vi "DataTreeCtrl unMountFile.vi"(8 "error in (no error)":errorcluster, 11 "DataTreeCtrl in":refnum<class "DataTreeCtrl.lvclass">) -> (0 "error out":errorcluster, 3 "DataTreeCtrl out":refnum<class "DataTreeCtrl.lvclass">)   [LabVIEW 2018, in "DataTreeCtrl.lvclass"]
uses:
  DataTreeCtrl.lvclass
  DataTreeCtrl.lvclass/DataTreeCtrl.ctl
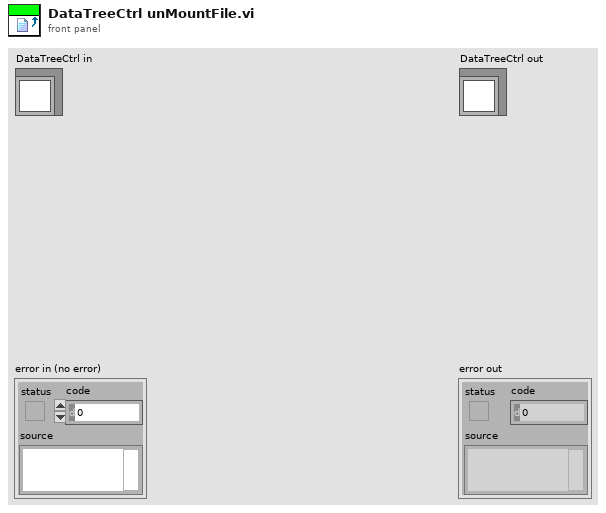
[diagram p1: front panel]
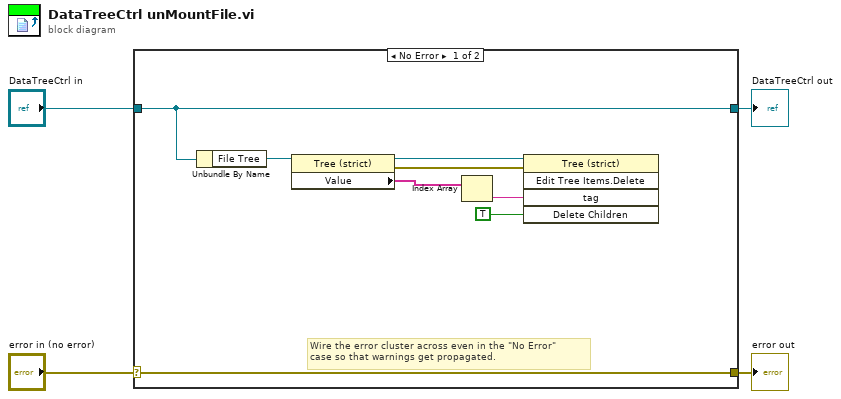
[diagram p0: block diagram]
diagram:
  n1 = case shown="No Error" "error in (no error)" {
    selector: "error in (no error)" -> [w12 w14]
    tunnel: [w12 w14] -> w3
    tunnel: [w10 w13] -> w1
    tunnel: "DataTreeCtrl in" -> [w10 w13]
    frame No Error {
      # "Wire the error cluster across even in the \"No Error\"\ncase so that warnings get propagated."
      n2 = Unbundle By Name(w10) -> ("File Tree"=w11:refnum<vi>)
      n3 = property class="Tree (strict)"(reference=w11) -> (reference out=w9:refnum<vi>, error out=w8:errorcluster, "Value"=w7:string[])  [unwired: 1 in]
      n4 = Index Array(array=w7) -> (element=w6:string)  [unwired: 1 in]
      n5 = invoke class="Tree (strict)" method="Edit Tree Items.Delete"(reference=w9, error in=w8, "tag"=w6, "Delete Children"=TRUE ("Delete Children?")) -> ()  [unwired: 1 in, 5 out]
    }
    frame Error {
    }
  }
  "error out" <- w3
  "DataTreeCtrl out" <- w1
